vi "test-TimeInterpBoolean-Test1.vi"() -> (3 "All tests passed":bool)   [LabVIEW 2019]
uses:
  <vilib>/Rock Robotics/WPI/ThirdParty/JAS_Junk/TrajLib/Rotation_CreateAngle.vi
  <vilib>/Rock Robotics/WPI/ThirdParty/JAS_Junk/TrajLib/Translation_Create.vi
  <vilib>/Rock Robotics/WPI/ThirdParty/JAS_Junk/TrajLib/Translation_Equals.vi
  <vilib>/Rock Robotics/WPI/ThirdParty/JAS_Junk/TrajLib/Rotation_Equals.vi
  <vilib>/Rock Robotics/WPI/ThirdParty/JAS_Junk/TrajLib/TimeInterpPose_CleanUp.vi
  <vilib>/Rock Robotics/WPI/ThirdParty/JAS_Junk/TrajLib/Util_CalcDist.vi
  <vilib>/gmath/interp.llb/Search Ordered Table.vi
  <vilib>/Rock Robotics/WPI/ThirdParty/JAS_Junk/TrajLib/Trajectory_Library.lvlib
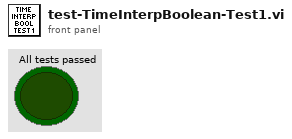
[diagram p1: front panel]
types:
  T1 = typedef "Trajectory_Library.lvlib/TIME_INTERPOLATABLE_BOOLEAN.ctl" = cluster{"TimeStamps":dbl[], "BooleanValue":bool[], "Min_TimeStamp":dbl, "Max_TimeStamp":dbl, "ItemCount":i32, "MaxBufferTime":dbl}
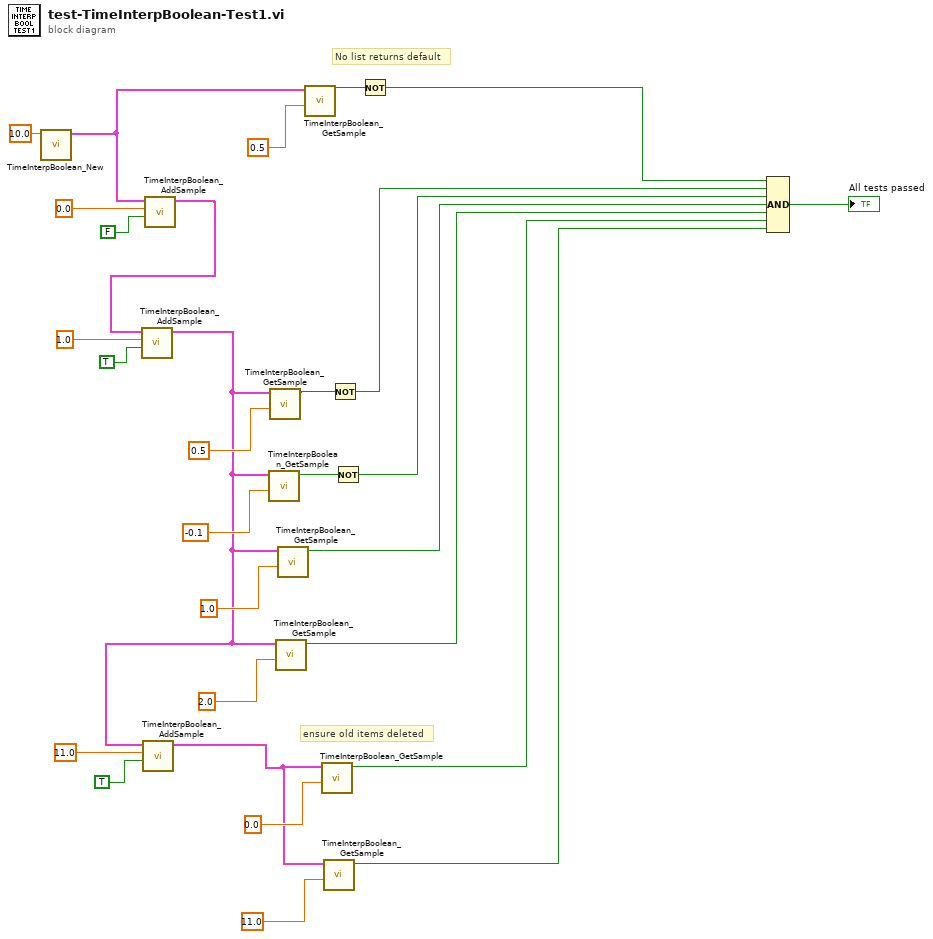
[diagram p0: block diagram]
diagram:
  # "ensure old items deleted"
  # "No list returns default"
  n1 = call <vilib>:"TimeInterpBoolean_New.vi"("MaxTime"=10.0) -> ("TimeInterpBoolean"=w22:T1)  [unwired: 10 in]
  n2 = call <vilib>:"TimeInterpBoolean_AddSample.vi"("Value"=FALSE, "TimeStamp"=0.0, "in TimeInterpBoolean"=w22) -> ("out TimeInterpBoolean"=w23:T1)  [unwired: 7 in, 1 out]
  n3 = call <vilib>:"TimeInterpBoolean_AddSample.vi"("Value"=TRUE, "TimeStamp"=1.0, "in TimeInterpBoolean"=w23) -> ("out TimeInterpBoolean"=w6:T1)  [unwired: 7 in, 1 out]
  n4 = call <vilib>:"TimeInterpBoolean_AddSample.vi"("Value"=TRUE, "TimeStamp"=11.0, "in TimeInterpBoolean"=w6) -> ("out TimeInterpBoolean"=w16:T1)  [unwired: 7 in, 1 out]
  n5 = call <vilib>:"TimeInterpBoolean_GetSample.vi"("TimeStamp"=-0.1, "TimeInterpBoolean"=w6) -> ("OutputBoolean"=w9:bool)  [unwired: 9 in]
  n6 = call <vilib>:"TimeInterpBoolean_GetSample.vi"("TimeStamp"=0.5, "TimeInterpBoolean"=w6) -> ("OutputBoolean"=w11:bool)  [unwired: 9 in]
  n7 = call <vilib>:"TimeInterpBoolean_GetSample.vi"("TimeStamp"=2.0, "TimeInterpBoolean"=w6) -> ("OutputBoolean"=w4:bool)  [unwired: 9 in]
  n8 = call <vilib>:"TimeInterpBoolean_GetSample.vi"("TimeStamp"=1.0, "TimeInterpBoolean"=w6) -> ("OutputBoolean"=w5:bool)  [unwired: 9 in]
  n9 = call <vilib>:"TimeInterpBoolean_GetSample.vi"("TimeStamp"=0.5, "TimeInterpBoolean"=w22) -> ("OutputBoolean"=w15:bool)  [unwired: 9 in]
  n10 = call <vilib>:"TimeInterpBoolean_GetSample.vi"("TimeStamp"=0.0, "TimeInterpBoolean"=w16) -> ("OutputBoolean"=w2:bool)  [unwired: 9 in]
  n11 = call <vilib>:"TimeInterpBoolean_GetSample.vi"("TimeStamp"=11.0, "TimeInterpBoolean"=w16) -> ("OutputBoolean"=w1:bool)  [unwired: 9 in]
  n12 = Not(x=w11) -> (.not. x?=w10:bool)
  n13 = Not(x=w9) -> (.not. x?=w8:bool)
  n14 = Not(x=w15) -> (.not. x?=w14:bool)
  n15 = Compound Arithmetic op=AND(w14, w10, w8, w5, w4, w2, w1) -> (→"All tests passed":bool)
